vi "Try Add Object Entry.vi"(8 "error in":errorcluster, 10 "Obj Entry":refnum<class "Object Entry.lvclass">, 11 "Obj Dict in":refnum<class "Object Dictionary.lvclass">) -> (0 "error out":errorcluster, 1 "Success":bool, 3 "Obj Dict out":refnum<class "Object Dictionary.lvclass">)   [LabVIEW 2020, in "CANopen.lvlib" / "Object Dictionary.lvclass"]
uses:
  Object Dictionary.lvclass
  Object Dictionary.lvclass/Object Dictionary.ctl
  Object Entry/Object Entry.lvclass
  Ordered-Dictionary/Ordered Object Dictionary/Source/Ordered Object Dictionary.lvclass
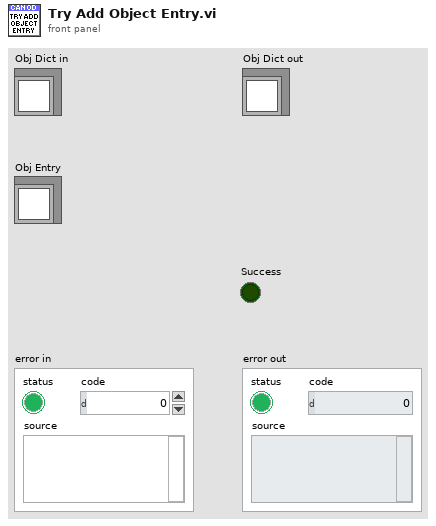
[diagram p1: front panel]
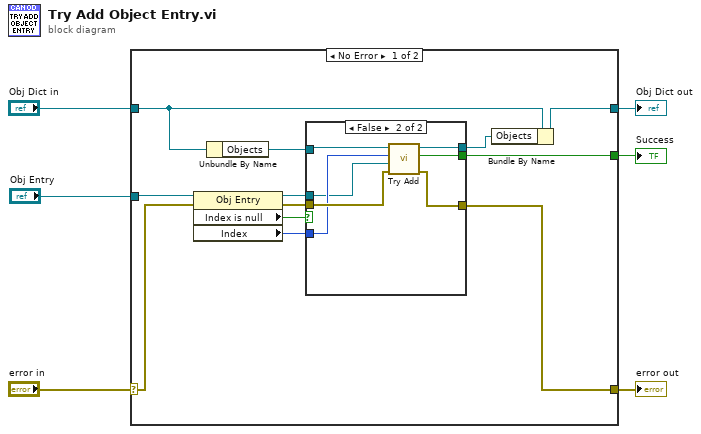
[diagram p0: block diagram]
diagram:
  n1 = case shown="No Error" "error in" {
    selector: "error in" -> [w15 w29]
    tunnel: [w9 w29] -> w3
    tunnel: [w8 w28] -> w5
    tunnel: "Obj Dict in" -> [w18 w28]
    tunnel: "Obj Entry" -> [w16 _]
    tunnel: [w13 _] -> w1
    frame No Error {
      n2 = property class="Obj Entry"(reference=w16, error in=w15) -> (reference out=w10:refnum<class "Object Entry.lvclass">, error out=w12:errorcluster, "Index is null"=w14:bool, "Index"=w11:u16)
      n3 = Unbundle By Name(w18) -> ("Objects"=w17:refnum<class "Ordered Object Dictionary.lvclass">)
      n4 = case shown="False" w14 {
        tunnel: w17 -> [w20 w27]
        tunnel: [_ w26] -> w13
        tunnel: w12 -> [w19 w25]
        tunnel: w11 -> [_ w24]
        tunnel: w10 -> [_ w23]
        tunnel: [w19 w22] -> w9
        tunnel: [w20 w21] -> w7
        frame True {
        }
        frame False {
          n5 = call "Try Add.vi"("error in"=w25, "Value"=w23, "Key"=w24, "Ordered Object Dictionary in"=w27) -> ("error out"=w22:errorcluster, "Success"=w26:bool, "Ordered Object Dictionary out"=w21:refnum<class "Ordered Object Dictionary.lvclass">)  [unwired: 5 in]
        }
      }
      n6 = Bundle By Name(cluster=w18, "Objects"=w7) -> (w8:refnum<class "Object Dictionary.lvclass">)
    }
    frame Error {
    }
  }
  "Obj Dict out" <- w5
  "error out" <- w3
  "Success" <- w1
